vi "Log on Error.vi"(7 "Logger Name":string, 8 "error in (no error)":errorcluster) -> (0 "error out":errorcluster)   [LabVIEW 2020, in "Global_logger.lvlib"]
uses:
  Global_logger.lvlib
  Levels.ctl
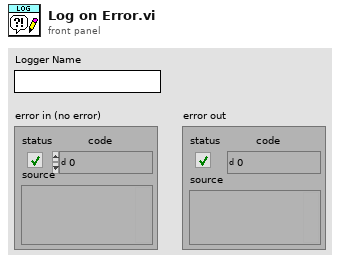
[diagram p1: front panel]
types:
  T1 = typedef "Global_logger.lvlib/Levels.ctl" = enum16{"ALL", "TRACE", "DEBUG", "INFO", "WARN", "ERROR", "FATAL", "OFF"}
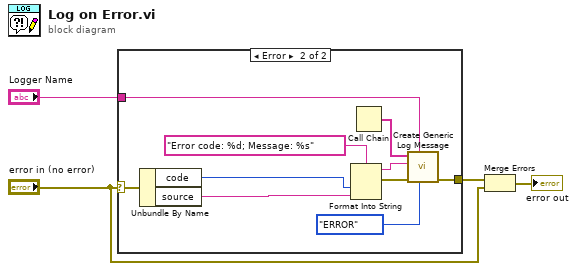
[diagram p0: block diagram]
diagram:
  n1 = case shown="Error" "error in (no error)" {
    selector: "error in (no error)" -> [w5 w8]
    tunnel: [w5 w14] -> w4
    tunnel: "Logger Name" -> [_ w6]
    frame No Error {
    }
    frame Error {
      n2 = Unbundle By Name(w8) -> ("code"=w13:i32, "source"=w12:string)
      n3 = Format Into String(format string="Error code: %d; Message: %s", w13, w12) -> (resulting string=w10:string, error out=w9:errorcluster)  [unwired: 2 in]
      n4 = Call Chain() -> (call chain=w15:string[])
      n5 = call "Create Generic Log Message.vi"("Level"=Levels."ERROR", "Logger Name"=w6, "error in (no error)"=w9, "Message"=w10, "Call Chain"=w15) -> ("error out"=w14:errorcluster)  [unwired: 6 in]
    }
  }
  n6 = Merge Errors(w4, "error in (no error)") -> (→"error out":errorcluster)
